vi "LvMPDC_SUB_ParseReplyString_LsInfo.vi"(10 "string":string="directory: musiclibrary/BlueOysterCult\ndirectory: musiclibrary/HeavyMetal\ndirectory: musiclibrary/Konan_2\nfile: musiclibrary/Konan_2/Everlasting.mp3\nLast-Modified: 2015-02-13T13:27:50Z\nTime: 221\nArtist: B'z\nTitle: Everlasting\nAlbum: KONAN BEST 2\nTrack: 1/15\nGenre: Jpop\nfile: musiclibrary/Konan_2/I can't stop my love for you.mp3\nLast-Modified: 2015-02-13T13:27:50Z\nTime: 258\nArtist: 愛内 里菜\nTitle: I can't stop my love for you\nAlbum: KONAN BEST 2\nTrack: 1/15\nGenre: Jpop\ndirectory: musiclibrary/Konan_3\ndirectory: musiclibrary/Konan_4\ndirectory: musiclibrary/Konan_X\n") -> (1 "file info[]":T2(array[cluster]) {"MusicInfo"."time" format="%<%H:%M:%S%3u>t"}, 2 "folder info[]":T2(array[cluster]) {"MusicInfo"."time" format="%<%H:%M:%S%3u>t"})   [LabVIEW 2012]
uses:
  LvMPDC_Typdef_MusicInfo.ctl
panel:
  # "directory: musiclibrary/BlueOysterCult\ndirectory: musiclibrary/HeavyMetal\ndirectory: musiclibrary/Konan_2\nfile: musiclibrary/Konan_2/Everlasting.mp3\nLast-Modified: 2015-02-13T13:27:50Z\nTime: 221\nArtist: B'z\nTitle: Everlasting\nAlbum: KONAN BEST 2\nTrack: 1/15\nGenre: Jpop\nfile: musiclibrary/Konan_2/I can't stop my love for you.mp3\nLast-Modified: 2015-02-13T13:27:50Z\nTime: 258\nArtist: 愛内 里菜\nTitle: I can't stop my love for you\nAlbum: KONAN BEST 2\nTrack: 1/15\nGenre: Jpop\ndirectory: musiclibrary/Konan_3\ndirectory: musiclibrary/Konan_4\ndirectory: musiclibrary/Konan_X"
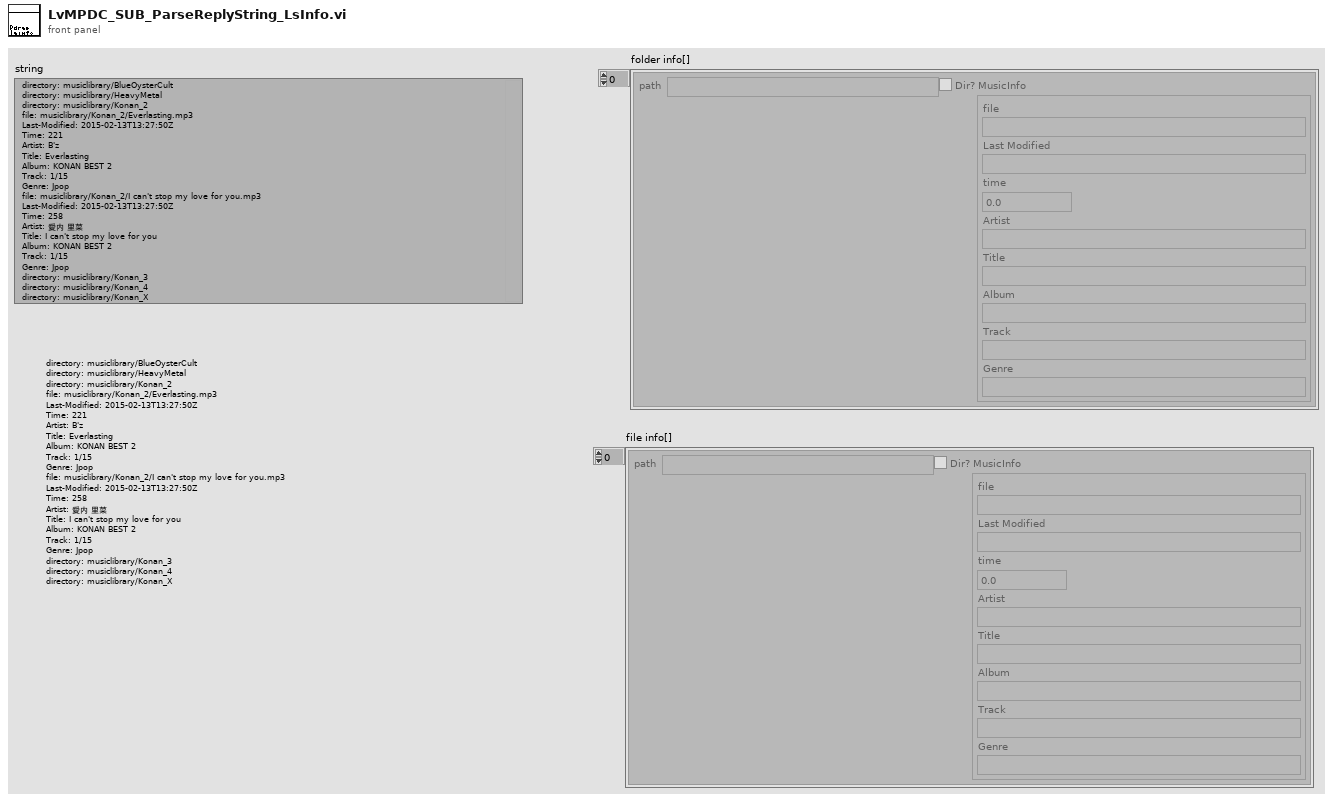
[diagram p1: front panel]
types:
  T1 = typedef "LvMPDC_Typdef_MusicInfo.ctl" = cluster{"file":string, "Last Modified":string, "time":dbl, "Artist":string, "Title":string, "Album":string, "Track":string, "Genre":string}
  T2 = cluster{"path":path, "Dir?":bool, "MusicInfo":T1}[]
  T3 = cluster{"path":path, "Dir?":bool, "MusicInfo":T1}
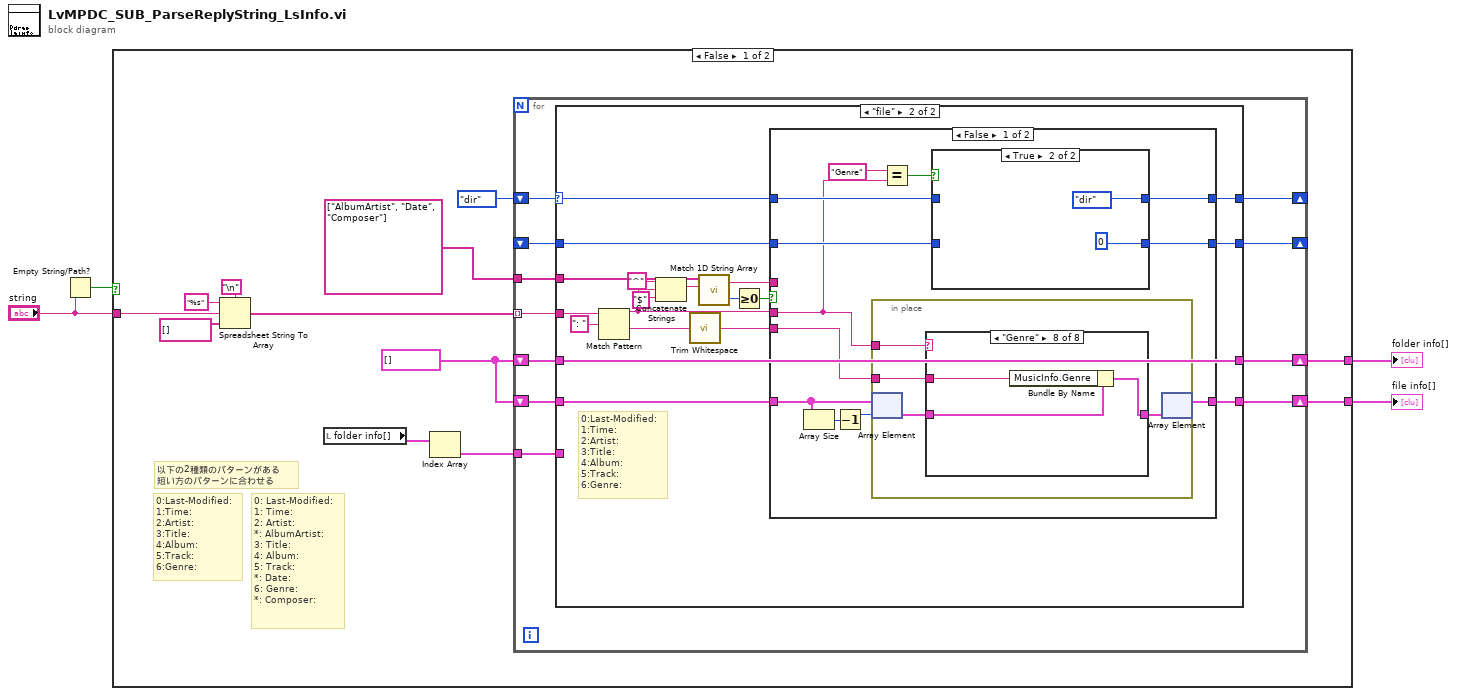
[diagram p0: block diagram]
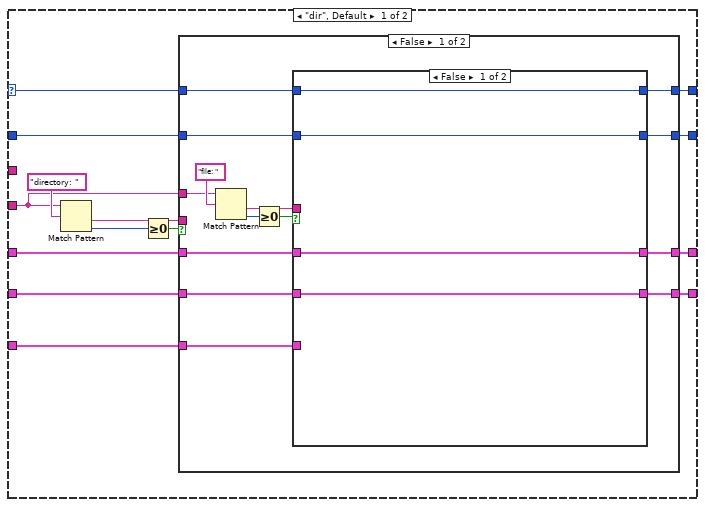
[diagram p2: hidden frame]
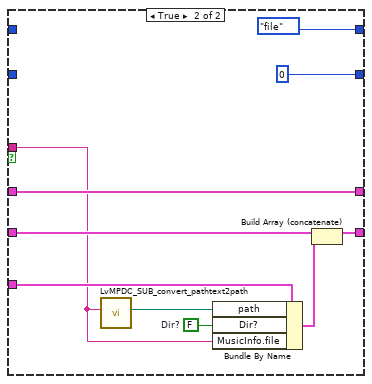
[diagram p3: hidden frame]
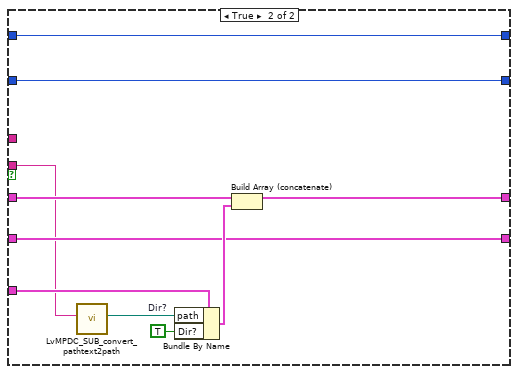
[diagram p4: hidden frame]
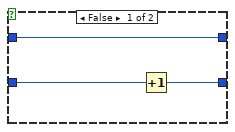
[diagram p5: hidden frame]
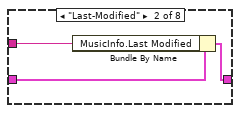
[diagram p7: hidden frame]
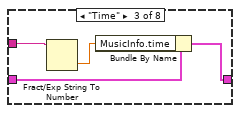
[diagram p8: hidden frame]
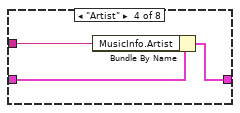
[diagram p9: hidden frame]
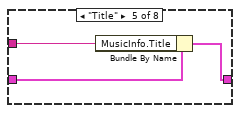
[diagram p10: hidden frame]
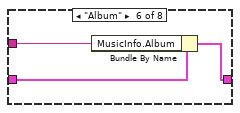
[diagram p11: hidden frame]
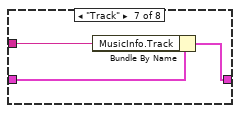
[diagram p12: hidden frame]
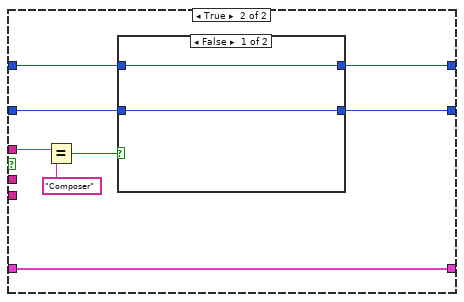
[diagram p13: hidden frame]
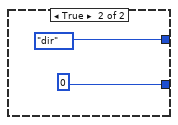
[diagram p14: hidden frame]
diagram:
  n1 = Empty String/Path?(string/path="string") -> (empty?=w3:bool)
  n2 = case shown="FALSE" w3 {
    tunnel: "string" -> [w13 _]
    tunnel: [w8 _] -> w2
    tunnel: [w6 _] -> w1
    frame False {
      w7 = T2 []
      # "以下の2種類のパターンがある\n短い方のパターンに合わせる"
      # "0:Last-Modified: \n1:Time: \n2:Artist: \n3:Title: \n4:Album: \n5:Track: \n6:Genre:"
      # "0: Last-Modified: \n1: Time: \n2: Artist: \n*: AlbumArtist: \n3: Title: \n4: Album: \n5: Track: \n*: Date: \n6: Genre: \n*: Composer:"
      n3 = Spreadsheet String To Array(delimiter (Tab)="\n", format string="%s" ("形式文字列"), spreadsheet string=w13, array type (2D Dbl)=string[] []) -> (array=w12:string[])
      n4 = local read "folder info[]"() -> (w10:T2)
      n5 = Index Array(array=w10) -> (element=w9:T3)  [unwired: 1 in]
      n6 = for {
        tunnel: w12 -> [w27] mode=indexing
        shift-right: [w23] -> _
        shift-left: enum16{"dir", "file"}."dir" ("status") -> [w26]
        shift-right: [w24] -> w8
        shift-left: w7 -> [w25]
        tunnel: w9 -> [w22]
        shift-right: [w21] -> _
        shift-left: _ -> [w20]
        shift-right: [w18] -> w6
        shift-left: w7 -> [w19]
        tunnel: string[] ["AlbumArtist", "Date", "Composer"] -> [w17]
        n7 = case shown="\"file\"" w26 {
          selector: w26 -> [w35 w92]
          tunnel: w27 -> [w32 w90]
          tunnel: [w37 w96] -> w24
          tunnel: w25 -> [w36 w96]
          tunnel: [w34 w91] -> w23
          tunnel: w22 -> [w33 _]
          tunnel: [w31 w97] -> w21
          tunnel: w20 -> [w30 w98]
          tunnel: w19 -> [w29 w95]
          tunnel: [w28 w94] -> w18
          tunnel: w17 -> [_ w88]
          frame "dir", Default {
            n8 = Match Pattern(string=w32, regular expression="directory: " ("正規表現")) -> (after substring=w40:string, offset past match=w39:i32)  [unwired: 1 in, 2 out]
            n9 = Greater Or Equal To 0?(x=w39) -> (x >= 0?=w38:bool)
            n10 = case shown="FALSE" w38 {
              tunnel: w40 -> [_ w71]
              tunnel: [w50 w79] -> w37
              tunnel: w36 -> [w51 w78]
              tunnel: w35 -> [w47 w77]
              tunnel: [w46 w77] -> w34
              tunnel: w33 -> [w49 w76]
              tunnel: w32 -> [w53 _]
              tunnel: [w45 w73] -> w31
              tunnel: w30 -> [w44 w73]
              tunnel: w29 -> [w43 w72]
              tunnel: [w42 w72] -> w28
              frame False {
                n11 = Match Pattern(string=w53, regular expression="file: " ("正規表現")) -> (after substring=w52:string, offset past match=w55:i32)  [unwired: 1 in, 2 out]
                n12 = Greater Or Equal To 0?(x=w55) -> (x >= 0?=w48:bool)
                n13 = case shown="FALSE" w48 {
                  tunnel: w52 -> [_ w61]
                  tunnel: w51 -> [w59 w65]
                  tunnel: [w59 w65] -> w50
                  tunnel: w49 -> [_ w68]
                  tunnel: w47 -> [w58 _]
                  tunnel: [w58 enum16{"dir", "file"}."file" ("status")] -> w46
                  tunnel: [w57 0] -> w45
                  tunnel: w44 -> [w57 _]
                  tunnel: w43 -> [w56 w64]
                  tunnel: [w56 w63] -> w42
                  frame False {
                  }
                  frame True {
                    w69 = FALSE  # Dir?
                    n14 = call "LvMPDC_SUB_convert_pathtext2path.vi"("pathtext"=w61) -> ("path"=w60:path)  [unwired: 10 in]
                    n15 = Bundle By Name(cluster=w68, "path"=w60, "Dir?"=w69, "MusicInfo.file"=w61) -> (w62:T3)
                    n16 = Build Array (concatenate)(w64, w62) -> (w63:T2)
                  }
                }
              }
              frame True {
                w75 = TRUE  # Dir?
                n17 = call "LvMPDC_SUB_convert_pathtext2path.vi"("pathtext"=w71) -> ("path"=w70:path)  [unwired: 10 in]
                n18 = Bundle By Name(cluster=w76, "path"=w70, "Dir?"=w75) -> (w74:T3)
                n19 = Build Array (concatenate)(w78, w74) -> (w79:T2)
              }
            }
          }
          frame "file" {
            # "0:Last-Modified: \n1:Time: \n2:Artist: \n3:Title: \n4:Album: \n5:Track: \n6:Genre:"
            n20 = Match Pattern(string=w90, regular expression=": ") -> (before substring=w80:string, after substring=w89:string)  [unwired: 1 in, 2 out]
            n21 = Concatenate Strings("^" ("文字列"), w80, "$") -> (w81:string)
            n22 = call <vilib>:"Trim Whitespace.vi"("string"=w89) -> ("trimmed string"=w93:string)  [unwired: 1 in]
            n23 = call <vilib>:"Match 1D String Array.vi"("Pattern"=w81, "Strings"=w88) -> ("index of element"=w87:i32, "Match"=w83:string)  [unwired: 2 in]
            n24 = Greater Or Equal To 0?(x=w87) -> (x >= 0?=w86:bool)
            n25 = case shown="FALSE" w86 {
              tunnel: w98 -> [w110 w145]
              tunnel: [w109 w143] -> w97
              tunnel: w95 -> [w108 w150]
              tunnel: [w107 w150] -> w94
              tunnel: w93 -> [w104 _]
              tunnel: w92 -> [w103 w146]
              tunnel: [w102 w144] -> w91
              tunnel: w83 -> [_ w148]
              tunnel: w80 -> [w99 _]
              frame False {
                n26 = Array Size(array=w108) -> (size(s)=w106:i32)
                n27 = Decrement(x=w106) -> (x-1=w105:i32)
                n28 = in-place {
                  in-place-border: w99 -> [w119]
                  in-place-border: w104 -> [w116]
                  n29 = in-place-array #1(w108, w105) -> (w118:T3)
                  n30 = case shown="\"Genre\"" w119 {
                    tunnel: w118 -> [w120 w123 w127 w130 w133 w136 w139 w142]
                    tunnel: [w120 w122 w126 w129 w132 w135 w138 w141] -> w117
                    tunnel: w116 -> [_ w121 w125 w128 w131 w134 w137 w140]
                    frame Default {
                    }
                    frame "Last-Modified" {
                      n31 = Bundle By Name(cluster=w123, "MusicInfo.Last Modified"=w121) -> (w122:T3)
                    }
                    frame "Time" {
                      n32 = Fract/Exp String To Number(string=w125) -> (number=w124:dbl)  [unwired: 3 in, 1 out]
                      n33 = Bundle By Name(cluster=w127, "MusicInfo.time"=w124) -> (w126:T3)
                    }
                    frame "Artist" {
                      n34 = Bundle By Name(cluster=w130, "MusicInfo.Artist"=w128) -> (w129:T3)
                    }
                    frame "Title" {
                      n35 = Bundle By Name(cluster=w133, "MusicInfo.Title"=w131) -> (w132:T3)
                    }
                    frame "Album" {
                      n36 = Bundle By Name(cluster=w136, "MusicInfo.Album"=w134) -> (w135:T3)
                    }
                    frame "Track" {
                      n37 = Bundle By Name(cluster=w139, "MusicInfo.Track"=w137) -> (w138:T3)
                    }
                    frame "Genre" {
                      n38 = Bundle By Name(cluster=w142, "MusicInfo.Genre"=w140) -> (w141:T3)
                    }
                  }
                  n39 = in-place-array #1(w117) -> (w107:T2)  [unwired: 1 out]
                }
                n40 = Equal?(x="Genre", y=w99) -> (x = y?=w100:bool)
                n41 = case shown="TRUE" w100 {
                  tunnel: w110 -> [w113 _]
                  tunnel: [w112 0] -> w109
                  tunnel: w103 -> [w111 _]
                  tunnel: [w111 enum16{"dir", "file"}."dir" ("status")] -> w102
                  frame False {
                    n42 = Increment(x=w113) -> (x+1=w112:i32)
                  }
                  frame True {
                  }
                }
              }
              frame True {
                n43 = Equal?(x=w148, y="Composer") -> (x = y?=w147:bool)
                n44 = case shown="FALSE" w147 {
                  tunnel: w146 -> [w152 _]
                  tunnel: w145 -> [w151 _]
                  tunnel: [w152 enum16{"dir", "file"}."dir" ("status")] -> w144
                  tunnel: [w151 0] -> w143
                  frame False {
                  }
                  frame True {
                  }
                }
              }
            }
          }
        }
      }
    }
    frame True {
    }
  }
  "folder info[]" <- w2
  "file info[]" <- w1
